vi "selector_compose_cmd.vi"(5 "Repeated Capability":string, 6 "Selector Name":string, 7 "Attribute":T1={"Identifier"="", "Descriptive Name"="", "Data Type"=enum."Integer 32", "Command"="", "Access"=enum."Read/Write", "Range Table"="", "Read Callback"="", "Write Callback"="", "Supported Models"="", "Instrument Options"="", "Index"=0, "OPC Wait"=FALSE, "No Status Check"=FALSE, "Cache Only"=FALSE}, 8 "error in":errorcluster caption="error in (no error)", 10 "Selector Attribute ID":string, 11 "VISA resource name":refnum<visa-resource-name>) -> (0 "error out":errorcluster, 2 "Attribute out":T1={"Identifier"="", "Descriptive Name"="", "Data Type"=enum."Integer 32", "Command"="", "Access"=enum."Read/Write", "Range Table"="", "Read Callback"="", "Write Callback"="", "Supported Models"="", "Instrument Options"="", "Index"=0, "OPC Wait"=FALSE, "No Status Check"=FALSE, "Cache Only"=FALSE}, 3 "VISA resource name out":refnum<visa-resource-name>)   [LabVIEW 2020, in "Rohde&Schwarz RTx Oscilloscopes.lvlib" / "rsidr_core.lvlib"]
uses:
  rsidr_core.lvlib
  type_Attribute.ctl
  type_Attribute_Data_Type.ctl
  type_ReadWriteAccess.ctl
  type_Error_Codes.ctl
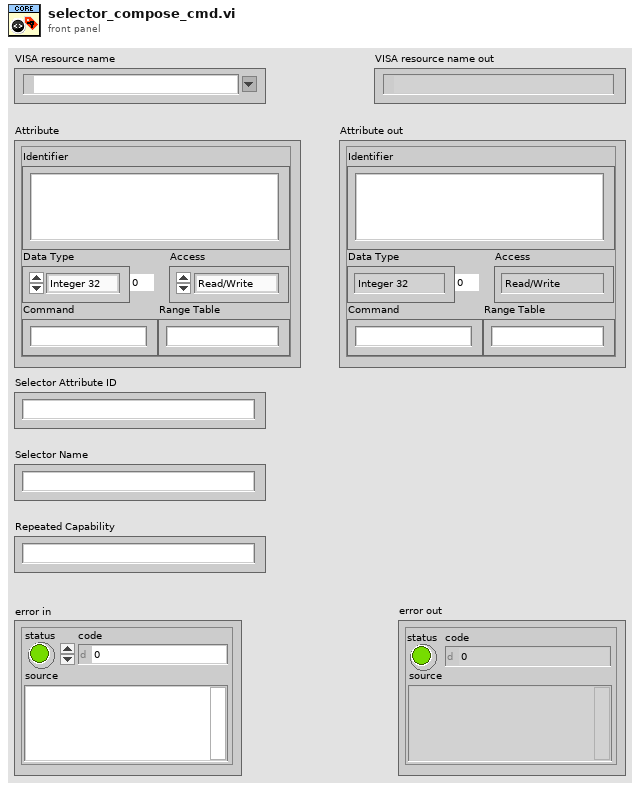
[diagram p1: front panel]
types:
  T1 = typedef "Rohde&Schwarz RTx Oscilloscopes.lvlib/rsidr_core.lvlib/type_Attribute.ctl" = cluster{"Identifier":string, "Descriptive Name":string, "Data Type":T2, "Command":string, "Access":T3, "Range Table":string, "Read Callback":string, "Write Callback":string, "Supported Models":string, "Instrument Options":string, "Index":i32, "OPC Wait":bool, "No Status Check":bool, "Cache Only":bool}
  T2 = typedef "Rohde&Schwarz RTx Oscilloscopes.lvlib/rsidr_core.lvlib/type_Attribute_Data_Type.ctl" = enum16{"Integer 32", "Double", "String", "Boolean", "None", "Integer 64", "RawString"}
  T3 = typedef "Rohde&Schwarz RTx Oscilloscopes.lvlib/rsidr_core.lvlib/type_ReadWriteAccess.ctl" = enum16{"Read Only", "Write Only", "Read/Write"}
  T4 = typedef "Rohde&Schwarz RTx Oscilloscopes.lvlib/rsidr_core.lvlib/type_Error_Codes.ctl" = enum16{"No_error", "VISA_err_ResourceNotFound", "VISA_err_Timeout", "VISA_warn_MoreDataAvailable", "RS_err_MissingCallback", "RS_err_InvalidAttribute", "RS_err_InvalidValue", "RS_err_UnknownResource", "RS_err_AlreadyInitialized", "RS_err_InstrumentStatus", "RS_err_BadRepCapName", "RS_err_TypesMismatch", "RS_err_ValueNotSupported", "RS_err_InvalidRngTable", "RS_err_IDqueryFail", "RS_err_UnexpResponse", "VISA_warn_ConfigNotLoaded", "RS_err_AttributeNotReadable", "RS_err_AttributeNotWritable", "RS_err_InstrumentType", "RS_err_InstrumentOption", "VISA_err_InvalidSize", "RS_err_ReliabilityIndicator", "VISA_warn_UnknownStatus", "VISA_warn_TermCharRead", "VISA_err_IO_error", "RS_err_FunctionNotSupported", "VISA_warn_QueueEmpty"}
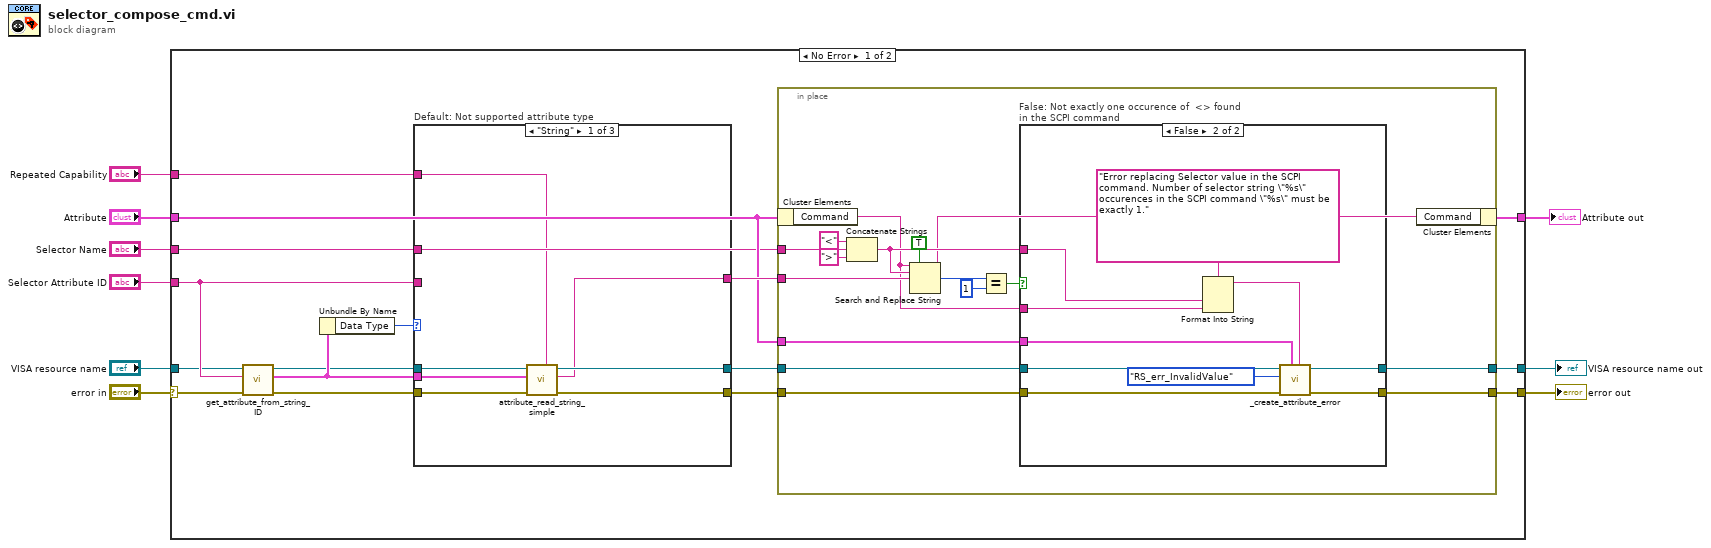
[diagram p0: block diagram]
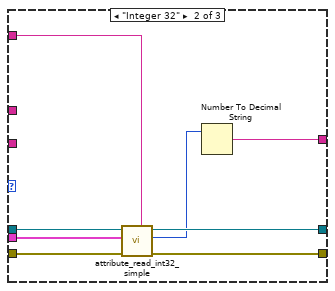
[diagram p3: hidden frame]
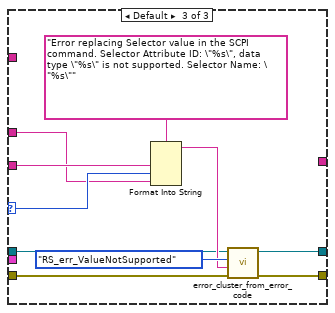
[diagram p4: hidden frame]
diagram:
  n1 = case shown="No Error" "error in" {
    selector: "error in" -> [w23 w81]
    tunnel: [w14 w79] -> w1
    tunnel: [w16 w81] -> w3
    tunnel: "VISA resource name" -> [w11 w80]
    tunnel: [w15 w80] -> w9
    tunnel: "Selector Attribute ID" -> [w24 _]
    tunnel: "Selector Name" -> [w12 _]
    tunnel: "Repeated Capability" -> [w20 _]
    tunnel: "Attribute" -> [w13 w79]
    frame No Error {
      n2 = call "get_attribute_from_string_ID.vi"("error in"=w23, "Attribute ID in"=w24, "VISA resource name"=w11) -> ("error out"=w22:errorcluster, "Attribute out"=w21:T1, "VISA resource name out"=w10:refnum<visa-resource-name>)  [unwired: 6 in]
      n3 = Unbundle By Name(w21) -> ("Data Type"=w25:T2)
      n4 = case "Default: Not supported attribute type" shown="\"String\"" w25 {
        selector: w25 -> [_ _ w70]
        tunnel: w22 -> [w60 w68 w73]
        tunnel: [w58 w66 w77] -> w17
        tunnel: w24 -> [_ _ w75]
        tunnel: w10 -> [w59 w67 w72]
        tunnel: w21 -> [w57 w65 _]
        tunnel: w20 -> [w56 w64 _]
        tunnel: [w55 w63 w71] -> w18
        tunnel: [w54 w61 _] -> w19
        tunnel: w12 -> [_ _ w69]
        frame "String" {
          n5 = call "attribute_read_string_simple.vi"("Repeated Capability"=w56, "Attribute"=w57, "error in"=w60, "VISA resource name"=w59) -> ("error out"=w58:errorcluster, "String out"=w54:string, "VISA resource name out"=w55:refnum<visa-resource-name>)  [unwired: 5 in]
        }
        frame "Integer 32" {
          n6 = call "attribute_read_int32_simple.vi"("Repeated Capability"=w64, "Attribute"=w65, "error in"=w68, "VISA resource name"=w67) -> ("error out"=w66:errorcluster, "Int32 out"=w62:i32, "VISA resource name out"=w63:refnum<visa-resource-name>)  [unwired: 5 in]
          n7 = Number To Decimal String(number=w62) -> (decimal integer string=w61:string)  [unwired: 1 in]
        }
        frame Default {
          n8 = Format Into String(format string="Error replacing Selector value in the SCPI command. Selector Attribute ID: \"%s\", data type \"%s\" is not supported. Selector Name: \"%s\"", w75, w70, w69) -> (resulting string=w74:string)  [unwired: 2 in, 1 out]
          n9 = call "error_cluster_from_error_code.vi"("error in"=w73, "Error Message (\"\")"=w74, "Error Enum in"=type_Error_Codes."RS_err_ValueNotSupported", "VISA resource name"=w72) -> ("error out"=w77:errorcluster, "VISA resource name out"=w71:refnum<visa-resource-name>)  [unwired: 6 in]
        }
      }
      n10 = in-place "In Place Element Structure" {
        in-place-border: w12 -> [w40]
        in-place-border: w19 -> [w37]
        in-place-border: w18 -> [w32]
        in-place-border: w17 -> [w31]
        in-place-border: [w30] -> w16
        in-place-border: [w29] -> w15
        in-place-border: w13 -> [w26]
        n11 = in-place-cluster #1 ("Unbundle / Bundle Elements")(w13) -> ("Command"=w28:string)
        n12 = Concatenate Strings("<", w40, ">") -> (w33:string)
        n13 = Search and Replace String(replace all?=TRUE ("replace all? (F)"), input string=w28, search string=w33, replace string=w37) -> (result string=w27:string, number of replacements=w36:i32)  [unwired: 4 in, 2 out]
        n14 = Equal?(x=w36, y=1) -> (x = y?=w34:bool)
        n15 = case "False: Not exactly one occurence of  <> found in the SCPI command" shown="False" w34 {
          tunnel: w31 -> [w42 w50]
          tunnel: [w42 w52] -> w30
          tunnel: w32 -> [w43 w49]
          tunnel: [w43 w48] -> w29
          tunnel: w33 -> [_ w47]
          tunnel: w28 -> [_ w46]
          tunnel: w26 -> [_ w45]
          frame True {
          }
          frame False {
            n16 = Format Into String(format string="Error replacing Selector value in the SCPI command. Number of selector string \"%s\" occurences in the SCPI command \"%s\" must be exactly 1.", w47, w46) -> (resulting string=w44:string)  [unwired: 2 in, 1 out]
            n17 = call "_create_attribute_error.vi"("Error Elaboration (\"\")"=w44, "Attribute"=w45, "error in"=w50, "Error Enum in"=type_Error_Codes."RS_err_InvalidValue", "VISA resource name"=w49) -> ("error out"=w52:errorcluster, "VISA resource name out"=w48:refnum<visa-resource-name>)  [unwired: 5 in]
          }
        }
        n18 = in-place-cluster #1 ("Unbundle / Bundle Elements")("Command"=w27) -> (w14:T1)
      }
    }
    frame Error {
    }
  }
  "error out" <- w3
  "VISA resource name out" <- w9
  "Attribute out" <- w1
